vi "Write access and modification time.vi"(8 "error in (no error)":errorcluster, 10 "access and modification time":T1, 11 "file attributes in":refnum<class "File Attributes.lvclass">) -> (0 "error out":errorcluster, 3 "file attributes out":refnum<class "File Attributes.lvclass">)   [LabVIEW 2020, in "NI_SFTP.lvlib" / "File Attributes.lvclass"]
doc: "Updates the access and modification time stored in this File Attributes object using LabVIEW timestamps. Due to limitations in the SFTP API, the access and modification time must be updated together."
uses:
  <vilib>/net/SFTP/File Attributes/File Attributes.lvclass
  <vilib>/net/SFTP/File Attributes/File Attributes.lvclass/File Attributes.ctl
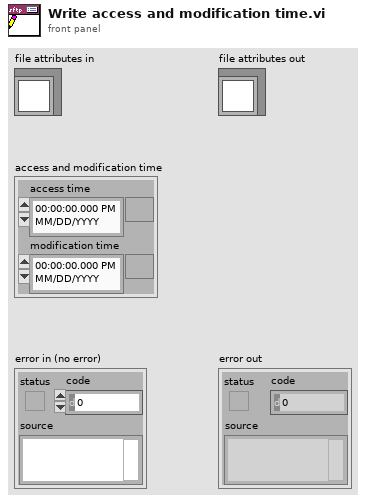
[diagram p1: front panel]
types:
  T1 = cluster{"access time":timestamp, "modification time":timestamp}
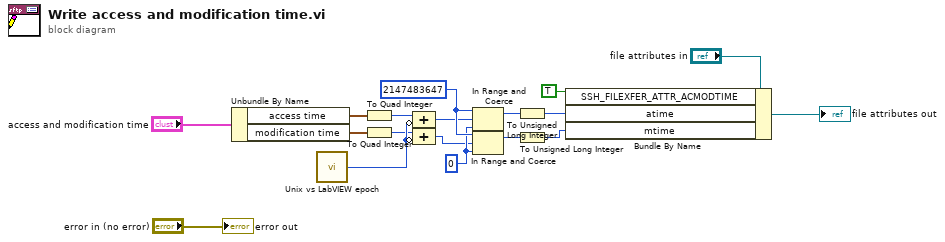
[diagram p0: block diagram]
diagram:
  w8 = i64 2147483647
  w7 = i64 0
  n1 = Unbundle By Name("access and modification time") -> ("access time"=w13:timestamp, "modification time"=w12:timestamp)
  n2 = call <vilib>:"Unix vs LabVIEW epoch.vi"() -> ("seconds from 1904-01-01 to 1970-01-01"=w10:i64)
  n3 = To Quad Integer(1:w13) -> (0:w11:i64)
  n4 = To Quad Integer(1:w12) -> (0:w9:i64)
  n5 = Compound Arithmetic op=ADD(w11, invert w10) -> (w3:i64)
  n6 = Compound Arithmetic op=ADD(w9, invert w10) -> (w4:i64)
  n7 = In Range and Coerce(upper limit=w8, x=w3, lower limit=w7) -> (coerced(x)=w6:i64)  [unwired: 1 out]
  n8 = In Range and Coerce(upper limit=w8, x=w4, lower limit=w7) -> (coerced(x)=w5:i64)  [unwired: 1 out]
  n9 = To Unsigned Long Integer(number=w6) -> (unsigned 32bit integer=w2:u32)
  n10 = To Unsigned Long Integer(number=w5) -> (unsigned 32bit integer=w1:u32)
  n11 = Bundle By Name(cluster="file attributes in", "SSH_FILEXFER_ATTR_ACMODTIME"=TRUE ("file attributes.SSH_FILEXFER_ATTR_ACMODTIME"), "atime"=w2, "mtime"=w1) -> (→"file attributes out":refnum<class "File Attributes.lvclass">)
  "error out" <- "error in (no error)"
